vi "S2C_OM8257_Poly_ReadTestDisplay.vi"(8 "Error In":errorcluster, 11 "Settings":T1={"Driver"="Omnia8257", "Command"="Read Test Display", "Return"="TestResult", "Parameters"="", "Timeout"=10.0}) -> (0 "Error Out":errorcluster, 3 "Response":string)   [LabVIEW 2015]
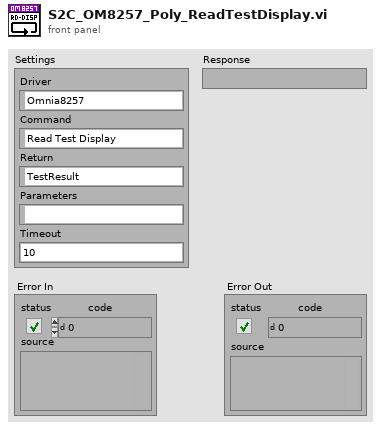
[diagram p1: front panel]
types:
  T1 = cluster{"Driver":string, "Command":string, "Return":string, "Parameters":string, "Timeout":dbl}
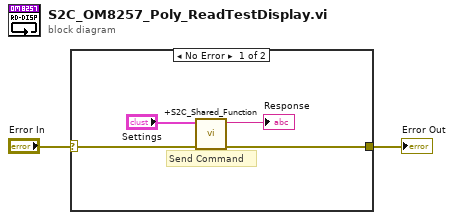
[diagram p0: block diagram]
diagram:
  n1 = case shown="No Error" "Error In" {
    selector: "Error In" -> [w4 w7]
    tunnel: [w6 w7] -> w1
    frame No Error {
      # "Send Command"
      n2 = call "+S2C_Shared_Function.vi"("Error In"=w4, "Settings"="Settings") -> ("Error Out"=w6:errorcluster, "Response"=→"Response":string)  [unwired: 8 in]
    }
    frame Error {
    }
  }
  "Error Out" <- w1
